vi "DriverStationGetData.vi"   [LabVIEW 2023]
doc: "This VI recieves data from the FRC 4265 Dashboard continuously, in all robot modes. These may include safety overrides, calibration commands, and configuration parameters. However this VI should never include standard driver or manipulator commands."
uses:
  f2972b46-d919-4210-bfdf-d3cf9c7f3ddc.vi
  GlobalDriverStationData.vi
  <vilib>/Rock Robotics/Network Tables/NT Read Number.vi
  <vilib>/Rock Robotics/Network Tables/NT Read Boolean.vi
  GlobalDrivebase.vi
  GlobalPoseAndTargeting.vi
  GlobalShooter.vi
  GlobalElevator.vi
  GlobalDriverStationCommands.vi
  GRNF_Joystick.vi
  <vilib>/Rock Robotics/Network Tables/NT Read Numeric Array.vi
  <vilib>/Rock Robotics/Network Tables/NT Read String.vi
  <vilib>/Utility/xml.llb/Write to XML File(string).vi
types:
  T1 = enum16{"Center", "North", "NorthWest", "West", "SouthWest", "South", "SouthEast", "East", "NorthEast"}
  T2 = typedef "WPI_JoystickDevRef.ctl" = cluster{"Device":T3}
  T3 = typedef "WPI_JoystickDeviceEnum.ctl" = enum16{"USB 0", "USB 1", "USB 2", "USB 3", "USB 4", "USB 5"}
  T4 = typedef "WPI_DriverStationAllianceInfo.ctl" = enum16{"Red", "Blue", "Invalid"}
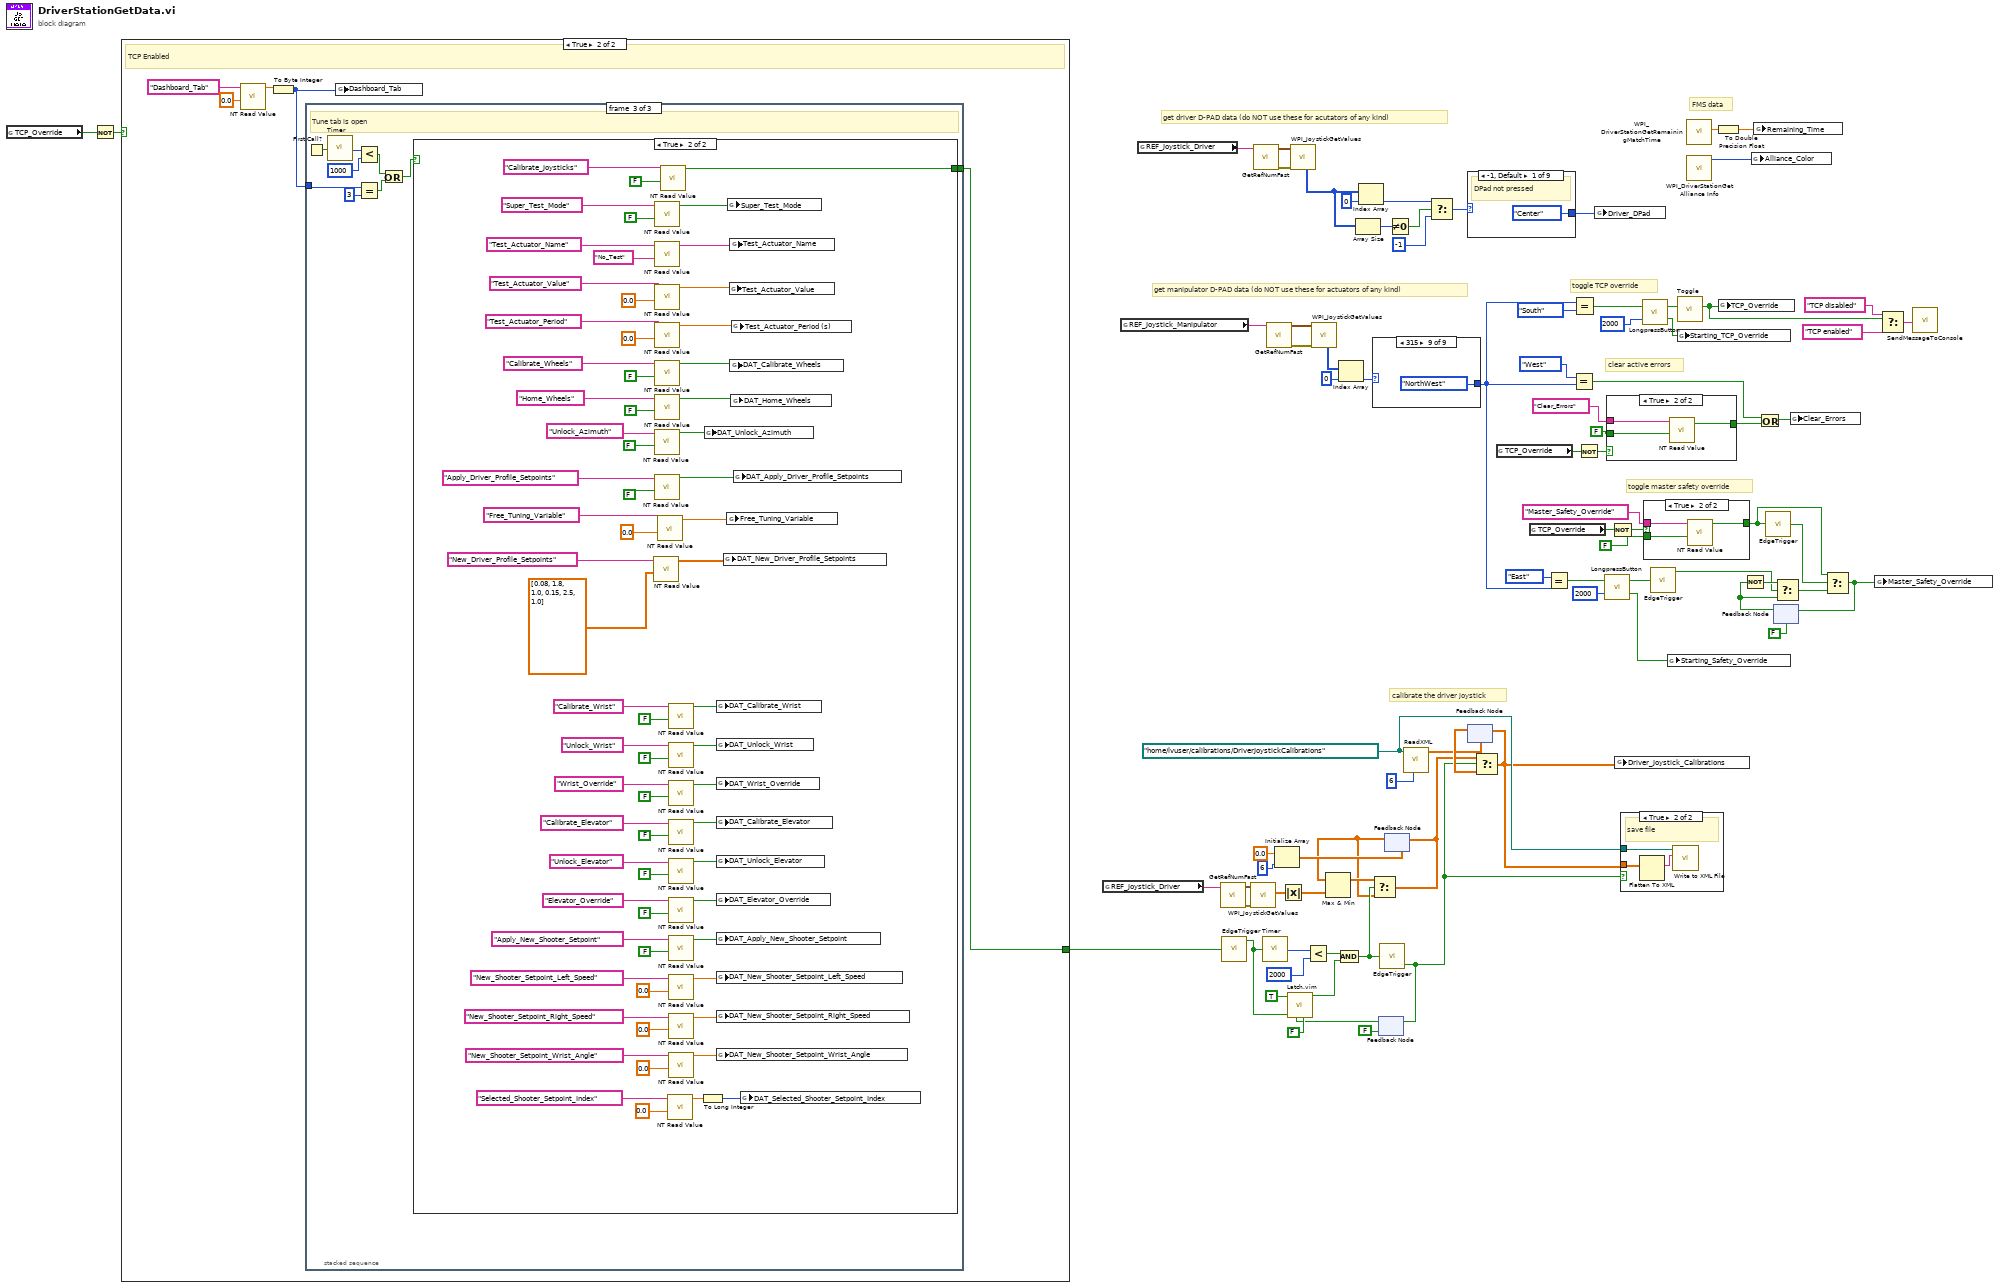
[diagram p0: block diagram]
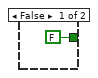
[diagram p2: hidden frame]
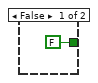
[diagram p3: hidden frame]
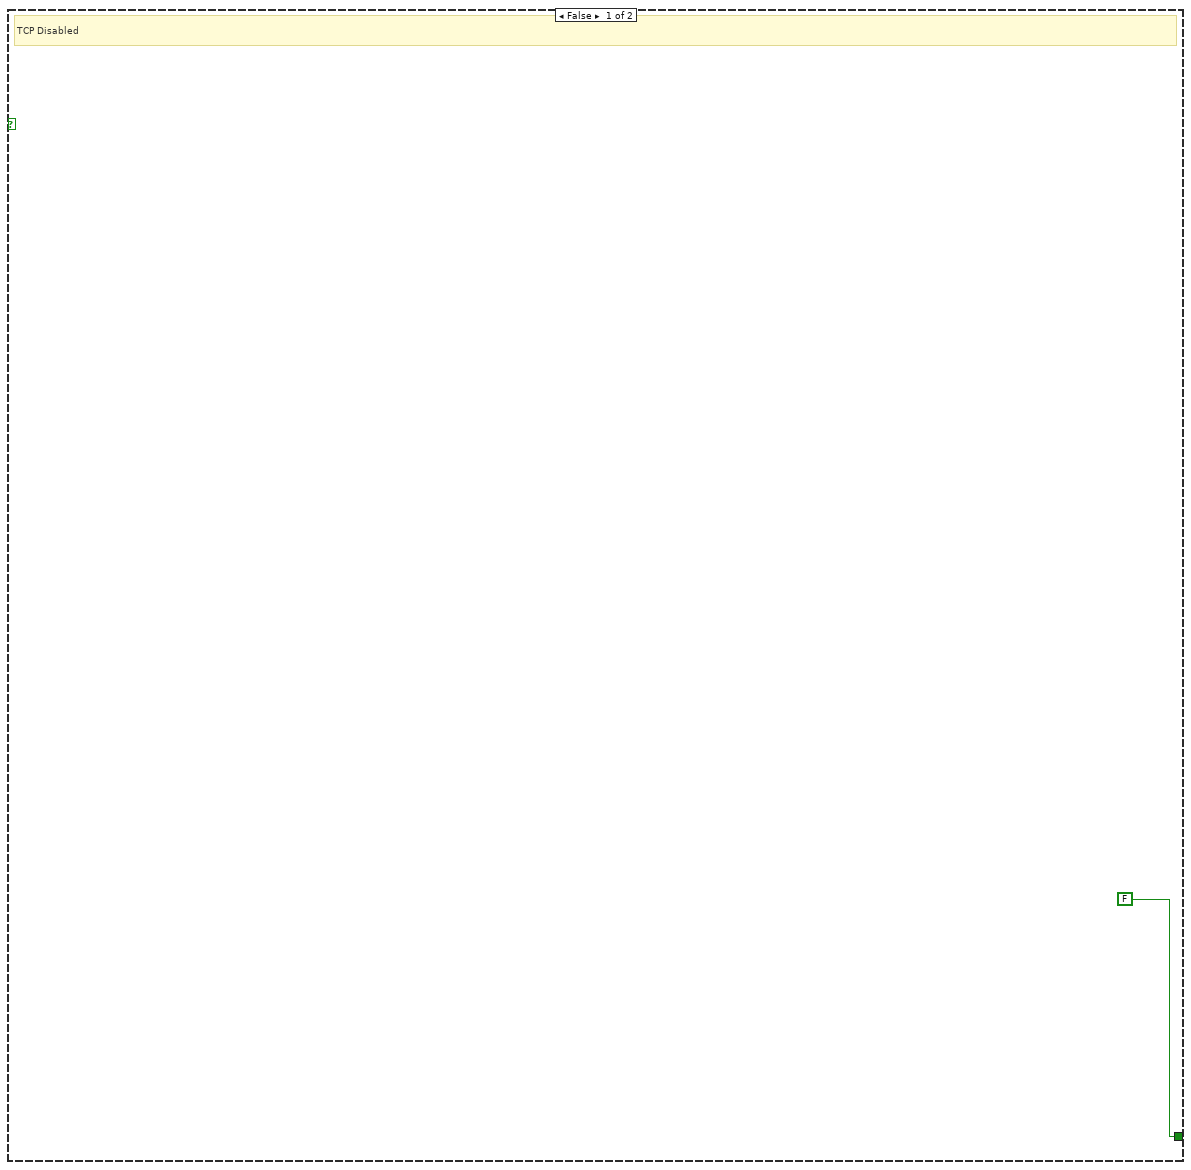
[diagram p4: hidden frame]
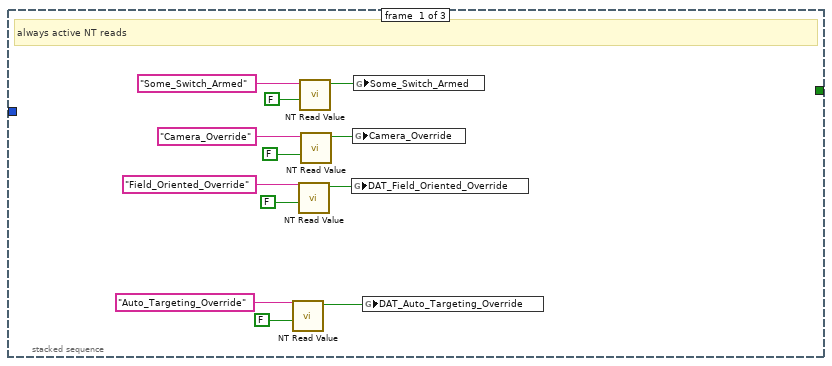
[diagram p5: hidden frame]
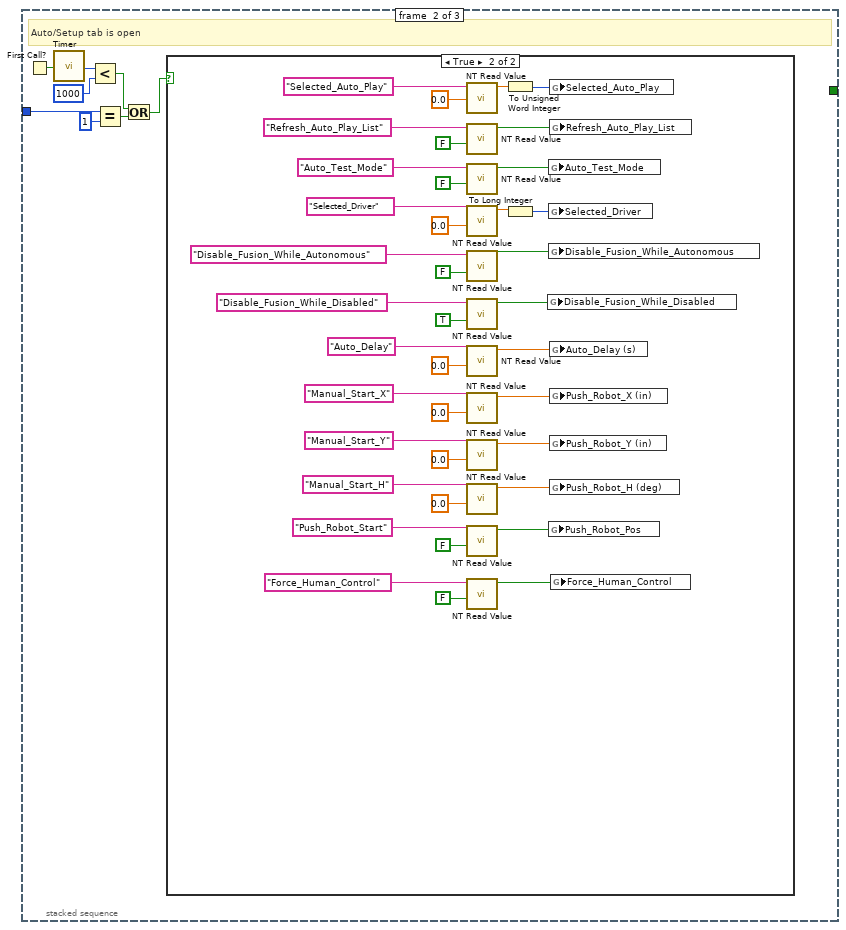
[diagram p6: hidden frame]
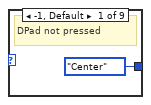
[diagram p9: hidden frame]
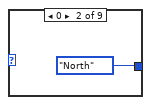
[diagram p10: hidden frame]
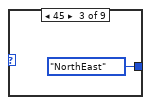
[diagram p11: hidden frame]
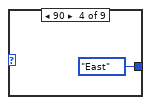
[diagram p12: hidden frame]
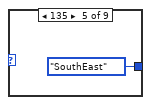
[diagram p13: hidden frame]
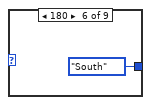
[diagram p14: hidden frame]
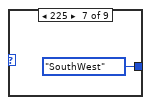
[diagram p15: hidden frame]
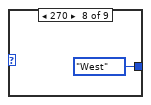
[diagram p16: hidden frame]
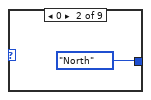
[diagram p17: hidden frame]
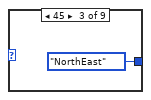
[diagram p18: hidden frame]
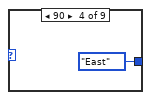
[diagram p19: hidden frame]
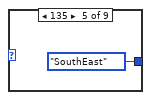
[diagram p20: hidden frame]
diagram:
  w82 = path "/home/lvuser/calibrations/DriverJoystickCalibrations" ("path")
  # "toggle master safety override"
  # "clear active errors"
  # "toggle TCP override"
  # "FMS data"
  # "get manipulator D-PAD data (do NOT use these for actuators of any kind)"
  # "get driver D-PAD data (do NOT use these for acutators of any kind)"
  # "calibrate the driver joystick"
  n1 = global read "GlobalDriverStationData.vi" "TCP_Override"() -> (w15:bool)
  n2 = Not(x=w15) -> (.not. x?=w14:bool)
  n3 = case shown="True" w14 {
    tunnel: [FALSE ("Boolean") w87] -> w26
    frame False {
      # "TCP Disabled"
    }
    frame True {
      # "TCP Enabled"
      n4 = call-poly <vilib>:"NT Read Value.vi"("default value"=0.0 ("Default Value"), "name"="Dashboard_Tab" ("refnum name")) -> ("value"=w89:dbl)  [unwired: 7 in, 2 out]
      n5 = To Byte Integer(number=w89) -> (8bit integer=w88:i8)
      n6 = stacked-sequence {
        tunnel: w88 -> [_ w111 w156]
        tunnel: [_ _ w154] -> w87
        frame #0 {
          # "always active NT reads"
          n7 = call-poly <vilib>:"NT Read Value.vi"("default value"=FALSE ("Default Value"), "name"="Auto_Targeting_Override" ("refnum name")) -> ("value"=w92:bool)  [unwired: 7 in, 2 out]
          n8 = call-poly <vilib>:"NT Read Value.vi"("default value"=FALSE ("Default Value"), "name"="Field_Oriented_Override" ("refnum name")) -> ("value"=w95:bool)  [unwired: 7 in, 2 out]
          n9 = call-poly <vilib>:"NT Read Value.vi"("default value"=FALSE ("Default Value"), "name"="Some_Switch_Armed" ("refnum name")) -> ("value"=w103:bool)  [unwired: 7 in, 2 out]
          n10 = call-poly <vilib>:"NT Read Value.vi"("default value"=FALSE ("Default Value"), "name"="Camera_Override" ("refnum name")) -> ("value"=w100:bool)  [unwired: 7 in, 2 out]
          n11 = global write "GlobalDrivebase.vi" "DAT_Field_Oriented_Override"(w95) -> ()
          n12 = global write "GlobalDriverStationData.vi" "Camera_Override"(w100) -> ()
          n13 = global write "GlobalDriverStationData.vi" "Some_Switch_Armed"(w103) -> ()
          n14 = global write "GlobalDrivebase.vi" "DAT_Auto_Targeting_Override"(w92) -> ()
        }
        frame #1 {
          # "Auto/Setup tab is open"
          n15 = First Call?() -> (First Call?: T/F=w109:bool)
          n16 = call "Timer.vi"("Reset Timer"=w109) -> ("Time (ms)"=w108:u32)
          n17 = Less?(x=w108, y=u32 1000 ("Time threshold (ms)")) -> (x < y?=w106:bool)
          n18 = Equal?(x=w111, y=i8 1) -> (x = y?=w107:bool)
          n19 = Or(x=w106, y=w107) -> (x .or. y?=w105:bool)
          n20 = case shown="True" w105 {
            frame False {
            }
            frame True {
              n21 = call-poly <vilib>:"NT Read Value.vi"("default value"=0.0 ("Default Value"), "name"="Selected_Auto_Play" ("refnum name")) -> ("value"=w138:dbl)  [unwired: 7 in, 2 out]
              n22 = call-poly <vilib>:"NT Read Value.vi"("default value"=FALSE ("Default Value"), "name"="Refresh_Auto_Play_List" ("refnum name")) -> ("value"=w137:bool)  [unwired: 7 in, 2 out]
              n23 = call-poly <vilib>:"NT Read Value.vi"("default value"=FALSE ("Default Value"), "name"="Auto_Test_Mode" ("refnum name")) -> ("value"=w149:bool)  [unwired: 7 in, 2 out]
              n24 = call-poly <vilib>:"NT Read Value.vi"("default value"=0.0 ("Default Value"), "name"="Selected_Driver" ("refnum name")) -> ("value"=w140:dbl)  [unwired: 7 in, 2 out]
              n25 = call-poly <vilib>:"NT Read Value.vi"("default value"=FALSE ("Default Value"), "name"="Disable_Fusion_While_Autonomous" ("refnum name")) -> ("value"=w143:bool)  [unwired: 7 in, 2 out]
              n26 = call-poly <vilib>:"NT Read Value.vi"("default value"=TRUE ("Default Value"), "name"="Disable_Fusion_While_Disabled" ("refnum name")) -> ("value"=w144:bool)  [unwired: 7 in, 2 out]
              n27 = call-poly <vilib>:"NT Read Value.vi"("default value"=0.0 ("Default Value"), "name"="Auto_Delay" ("refnum name")) -> ("value"=w142:dbl)  [unwired: 7 in, 2 out]
              n28 = call-poly <vilib>:"NT Read Value.vi"("default value"=0.0 ("Default Value"), "name"="Manual_Start_X" ("refnum name")) -> ("value"=w145:dbl)  [unwired: 7 in, 2 out]
              n29 = call-poly <vilib>:"NT Read Value.vi"("default value"=0.0 ("Default Value"), "name"="Manual_Start_Y" ("refnum name")) -> ("value"=w146:dbl)  [unwired: 7 in, 2 out]
              n30 = call-poly <vilib>:"NT Read Value.vi"("default value"=0.0 ("Default Value"), "name"="Manual_Start_H" ("refnum name")) -> ("value"=w147:dbl)  [unwired: 7 in, 2 out]
              n31 = call-poly <vilib>:"NT Read Value.vi"("default value"=FALSE ("Default Value"), "name"="Push_Robot_Start" ("refnum name")) -> ("value"=w148:bool)  [unwired: 7 in, 2 out]
              n32 = call-poly <vilib>:"NT Read Value.vi"("default value"=FALSE ("Default Value"), "name"="Force_Human_Control" ("refnum name")) -> ("value"=w114:bool)  [unwired: 7 in, 2 out]
              n33 = To Unsigned Word Integer(number=w138) -> (unsigned 16bit integer=w139:u16)
              n34 = To Long Integer(number=w140) -> (32bit integer=w141:i32)
              n35 = global write "GlobalDriverStationData.vi" "Disable_Fusion_While_Disabled"(w144) -> ()
              n36 = global write "GlobalDriverStationData.vi" "Auto_Test_Mode"(w149) -> ()
              n37 = global write "GlobalDriverStationData.vi" "Selected_Driver"(w141) -> ()
              n38 = global write "GlobalDriverStationData.vi" "Disable_Fusion_While_Autonomous"(w143) -> ()
              n39 = global write "GlobalPoseAndTargeting.vi" "Push_Robot_Pos"(w148) -> ()
              n40 = global write "GlobalDriverStationData.vi" "Selected_Auto_Play"(w139) -> ()
              n41 = global write "GlobalDriverStationData.vi" "Refresh_Auto_Play_List"(w137) -> ()
              n42 = global write "GlobalDriverStationData.vi" "Auto_Delay (s)"(w142) -> ()
              n43 = global write "GlobalPoseAndTargeting.vi" "Push_Robot_X (in)"(w145) -> ()
              n44 = global write "GlobalPoseAndTargeting.vi" "Push_Robot_Y (in)"(w146) -> ()
              n45 = global write "GlobalPoseAndTargeting.vi" "Push_Robot_H (deg)"(w147) -> ()
              n46 = global write "GlobalDriverStationData.vi" "Force_Human_Control"(w114) -> ()
            }
          }
        }
        frame #2 {
          # "Tune tab is open"
          n47 = First Call?() -> (First Call?: T/F=w153:bool)
          n48 = call "Timer.vi"("Reset Timer"=w153) -> ("Time (ms)"=w152:u32)
          n49 = Less?(x=w152, y=u32 1000 ("Time threshold (ms)")) -> (x < y?=w150:bool)
          n50 = Equal?(x=w156, y=i8 3) -> (x = y?=w158:bool)
          n51 = Or(x=w150, y=w158) -> (x .or. y?=w155:bool)
          n52 = case shown="True" w155 {
            tunnel: [_ w200] -> w154
            frame False {
            }
            frame True {
              n53 = call-poly <vilib>:"NT Read Value.vi"("default value"=dbl[] [0.08, 1.8, 1.0, 0.15, 2.5, 1.0] ("Default Value"), "name"="New_Driver_Profile_Setpoints" ("Name")) -> ("value"=w196:dbl[])  [unwired: 7 in, 2 out]
              n54 = call-poly <vilib>:"NT Read Value.vi"("default value"=FALSE ("Default Value"), "name"="Unlock_Azimuth" ("refnum name")) -> ("value"=w193:bool)  [unwired: 7 in, 2 out]
              n55 = call-poly <vilib>:"NT Read Value.vi"("default value"=FALSE ("Default Value"), "name"="Apply_Driver_Profile_Setpoints" ("Name")) -> ("value"=w197:bool)  [unwired: 7 in, 2 out]
              n56 = call-poly <vilib>:"NT Read Value.vi"("default value"=FALSE ("Default Value"), "name"="Super_Test_Mode" ("refnum name")) -> ("value"=w225:bool)  [unwired: 7 in, 2 out]
              n57 = call-poly <vilib>:"NT Read Value.vi"("default value"="No_Test" ("Default Value"), "name"="Test_Actuator_Name" ("refnum name")) -> ("value"=w220:string)  [unwired: 7 in, 2 out]
              n58 = call-poly <vilib>:"NT Read Value.vi"("default value"=0.0 ("Default Value"), "name"="Test_Actuator_Value" ("refnum name")) -> ("value"=w221:dbl)  [unwired: 7 in, 2 out]
              n59 = call-poly <vilib>:"NT Read Value.vi"("default value"=0.0 ("Default Value"), "name"="Test_Actuator_Period" ("refnum name")) -> ("value"=w222:dbl)  [unwired: 7 in, 2 out]
              n60 = call-poly <vilib>:"NT Read Value.vi"("default value"=FALSE ("Default Value"), "name"="Calibrate_Wheels" ("refnum name")) -> ("value"=w199:bool)  [unwired: 7 in, 2 out]
              n61 = call-poly <vilib>:"NT Read Value.vi"("default value"=FALSE ("Default Value"), "name"="Home_Wheels" ("refnum name")) -> ("value"=w198:bool)  [unwired: 7 in, 2 out]
              n62 = call-poly <vilib>:"NT Read Value.vi"("default value"=0.0 ("Default Value"), "name"="Free_Tuning_Variable" ("refnum name")) -> ("value"=w206:dbl)  [unwired: 7 in, 2 out]
              n63 = call-poly <vilib>:"NT Read Value.vi"("default value"=FALSE ("Default Value"), "name"="Calibrate_Joysticks" ("refnum name")) -> ("value"=w200:bool)  [unwired: 7 in, 2 out]
              n64 = call-poly <vilib>:"NT Read Value.vi"("default value"=0.0, "name"="Selected_Shooter_Setpoint_Index" ("refnum name")) -> ("value"=w160:dbl)  [unwired: 7 in, 2 out]
              n65 = call-poly <vilib>:"NT Read Value.vi"("default value"=FALSE ("Default Value"), "name"="Calibrate_Wrist" ("refnum name")) -> ("value"=w190:bool)  [unwired: 7 in, 2 out]
              n66 = call-poly <vilib>:"NT Read Value.vi"("default value"=FALSE ("Default Value"), "name"="Unlock_Wrist" ("refnum name")) -> ("value"=w180:bool)  [unwired: 7 in, 2 out]
              n67 = call-poly <vilib>:"NT Read Value.vi"("default value"=FALSE ("Default Value"), "name"="Wrist_Override" ("refnum name")) -> ("value"=w175:bool)  [unwired: 7 in, 2 out]
              n68 = call-poly <vilib>:"NT Read Value.vi"("default value"=FALSE ("Default Value"), "name"="Calibrate_Elevator" ("refnum name")) -> ("value"=w187:bool)  [unwired: 7 in, 2 out]
              n69 = call-poly <vilib>:"NT Read Value.vi"("default value"=FALSE ("Default Value"), "name"="Unlock_Elevator" ("refnum name")) -> ("value"=w186:bool)  [unwired: 7 in, 2 out]
              n70 = call-poly <vilib>:"NT Read Value.vi"("default value"=FALSE ("Default Value"), "name"="Elevator_Override" ("refnum name")) -> ("value"=w181:bool)  [unwired: 7 in, 2 out]
              n71 = call-poly <vilib>:"NT Read Value.vi"("default value"=FALSE ("Default Value"), "name"="Apply_New_Shooter_Setpoint" ("refnum name")) -> ("value"=w172:bool)  [unwired: 7 in, 2 out]
              n72 = call-poly <vilib>:"NT Read Value.vi"("default value"=0.0, "name"="New_Shooter_Setpoint_Left_Speed" ("refnum name")) -> ("value"=w171:dbl)  [unwired: 7 in, 2 out]
              n73 = call-poly <vilib>:"NT Read Value.vi"("default value"=0.0, "name"="New_Shooter_Setpoint_Right_Speed" ("refnum name")) -> ("value"=w168:dbl)  [unwired: 7 in, 2 out]
              n74 = call-poly <vilib>:"NT Read Value.vi"("default value"=0.0, "name"="New_Shooter_Setpoint_Wrist_Angle" ("refnum name")) -> ("value"=w167:dbl)  [unwired: 7 in, 2 out]
              n75 = To Long Integer(number=w160) -> (32bit integer=w159:i32)
              n76 = global write "GlobalDrivebase.vi" "DAT_Unlock_Azimuth"(w193) -> ()
              n77 = global write "GlobalShooter.vi" "DAT_Calibrate_Wrist"(w190) -> ()
              n78 = global write "GlobalShooter.vi" "DAT_Unlock_Wrist"(w180) -> ()
              n79 = global write "GlobalShooter.vi" "DAT_Wrist_Override"(w175) -> ()
              n80 = global write "GlobalElevator.vi" "DAT_Calibrate_Elevator"(w187) -> ()
              n81 = global write "GlobalElevator.vi" "DAT_Unlock_Elevator"(w186) -> ()
              n82 = global write "GlobalElevator.vi" "DAT_Elevator_Override"(w181) -> ()
              n83 = global write "GlobalShooter.vi" "DAT_Apply_New_Shooter_Setpoint"(w172) -> ()
              n84 = global write "GlobalShooter.vi" "DAT_New_Shooter_Setpoint_Left_Speed"(w171) -> ()
              n85 = global write "GlobalShooter.vi" "DAT_New_Shooter_Setpoint_Right_Speed"(w168) -> ()
              n86 = global write "GlobalShooter.vi" "DAT_New_Shooter_Setpoint_Wrist_Angle"(w167) -> ()
              n87 = global write "GlobalDrivebase.vi" "DAT_New_Driver_Profile_Setpoints"(w196) -> ()
              n88 = global write "GlobalDriverStationData.vi" "Free_Tuning_Variable"(w206) -> ()
              n89 = global write "GlobalDriverStationData.vi" "Super_Test_Mode"(w225) -> ()
              n90 = global write "GlobalDriverStationData.vi" "Test_Actuator_Value"(w221) -> ()
              n91 = global write "GlobalDriverStationData.vi" "Test_Actuator_Name"(w220) -> ()
              n92 = global write "GlobalDrivebase.vi" "DAT_Calibrate_Wheels"(w199) -> ()
              n93 = global write "GlobalDrivebase.vi" "DAT_Home_Wheels"(w198) -> ()
              n94 = global write "GlobalDriverStationData.vi" "Test_Actuator_Period (s)"(w222) -> ()
              n95 = global write "GlobalDrivebase.vi" "DAT_Apply_Driver_Profile_Setpoints"(w197) -> ()
              n96 = global write "GlobalShooter.vi" "DAT_Selected_Shooter_Setpoint_Index"(w159) -> ()
            }
          }
        }
      }
      n97 = global write "GlobalDriverStationData.vi" "Dashboard_Tab"(w88) -> ()
    }
  }
  n98 = global read "GlobalDriverStationCommands.vi" "REF_Joystick_Driver"() -> (w7:string)
  n99 = global read "GlobalDriverStationCommands.vi" "REF_Joystick_Manipulator"() -> (w8:string)
  n100 = global read "GlobalDriverStationCommands.vi" "REF_Joystick_Driver"() -> (w9:string)
  n101 = call-poly "GetRefNumFast.vi"("RefNum Name"=w7) -> ("Error"=w77:errorcluster, "Device Reference"=w78:T2)  [unwired: 5 in]
  n102 = call "EdgeTrigger.vi"("Input Signal"=w26) -> ("Rising Edge Trigger"=w76:bool)  [unwired: 2 out]
  n103 = call <vilib>:"WPI_JoystickGetValues.vi"("error in (no error)"=w77, "JoystickDevRef"=w78) -> ("Axes"=w66:dbl[])  [unwired: 5 in, 4 out]
  n104 = call-poly "GetRefNumFast.vi"("RefNum Name"=w9) -> ("Error"=w56:errorcluster, "Device Reference"=w57:T2)  [unwired: 5 in]
  n105 = call "Timer.vi"("Reset Timer"=w76) -> ("Time (ms)"=w80:u32)
  n106 = call-poly "GetRefNumFast.vi"("RefNum Name"=w8) -> ("Error"=w84:errorcluster, "Device Reference"=w85:T2)  [unwired: 5 in]
  n107 = Initialize Array(0.0 ("element"), 6 ("dimension size")) -> (w59:dbl[])
  n108 = Absolute Value(x=w66) -> (abs(x)=w63:dbl[])
  n109 = call <vilib>:"WPI_JoystickGetValues.vi"("error in (no error)"=w56, "JoystickDevRef"=w57) -> ("POVs"=w6:i16[])  [unwired: 5 in, 4 out]
  n110 = Less?(x=w80, y=u32 2000) -> (x < y?=w73:bool)
  n111 = call <vilib>:"WPI_JoystickGetValues.vi"("error in (no error)"=w84, "JoystickDevRef"=w85) -> ("POVs"=w51:i16[])  [unwired: 5 in, 4 out]
  n112 = Index Array(array=w51, index=0) -> (element=w52:i16)
  n113 = Array Size(array=w6) -> (size(s)=w5:i32)
  n114 = Index Array(array=w6, index=0) -> (element=w4:i16)
  n115 = case shown="315" w52 {
    tunnel: [T1."Center" T1."North" T1."NorthEast" T1."East" T1."SouthEast" T1."South" T1."SouthWest" T1."West" T1."NorthWest"] -> w24
    frame -1, Default {
      # "DPad not pressed"
    }
    frame 0 {
    }
    frame 45 {
    }
    frame 90 {
    }
    frame 135 {
    }
    frame 180 {
    }
    frame 225 {
    }
    frame 270 {
    }
    frame 315 {
    }
  }
  n116 = feedback #1(FALSE ("Falling Edge Trigger")) -> (w70:bool)
  n117 = call "Latch.vim"("Default Value"=FALSE, "Reset"=w70, "Latch Signal"=w76, "Latch Value"=TRUE) -> ("Latched"=w72:bool)  [unwired: 7 in]
  n118 = And(x=w73, y=w72) -> (x .and. y?=w71:bool)
  n119 = call "EdgeTrigger.vi"("Input Signal"=w71) -> ("Falling Edge Trigger"=w68:bool)  [unwired: 2 out]
  n120 = feedback-in #1(w68) -> ()
  n121 = feedback #2(w59) -> (w58:dbl[])
  n122 = Max & Min(x=w58, y=w63) -> (max(x,y)=w65:dbl[])  [unwired: 1 out]
  n123 = Select(t=w65, s=w71, f=w58) -> (s? t:f=w64:dbl[])
  n124 = feedback-in #2(w64) -> ()
  n125 = Not Equal To 0?(x=w5) -> (x != 0?=w3:bool)
  n126 = call "ReadXML.vi"("Default Number of Elements"=6, "File Path (.xml)"=w82) -> ("Data"=w81:dbl[])  [unwired: 8 in, 1 out]
  n127 = Select(t=w4, s=w3, f=i16 -1) -> (s? t:f=w2:i16)
  n128 = case shown="-1, Default" w2 {
    tunnel: [T1."Center" T1."North" T1."NorthEast" T1."East" T1."SouthEast" T1."South" T1."SouthWest" T1."West" T1."NorthWest"] -> w54
    frame -1, Default {
      # "DPad not pressed"
    }
    frame 0 {
    }
    frame 45 {
    }
    frame 90 {
    }
    frame 135 {
    }
    frame 180 {
    }
    frame 225 {
    }
    frame 270 {
    }
    frame 315 {
    }
  }
  n129 = feedback #3(w81) -> (w83:dbl[])
  n130 = Select(t=w64, s=w68, f=w83) -> (s? t:f=w67:dbl[])
  n131 = feedback-in #3(w67) -> ()
  n132 = global read "GlobalDriverStationData.vi" "TCP_Override"() -> (w11:bool)
  n133 = global read "GlobalDriverStationData.vi" "TCP_Override"() -> (w13:bool)
  n134 = Equal?(x=T1."East", y=w24) -> (x = y?=w40:bool)
  n135 = Equal?(x=T1."West", y=w24) -> (x = y?=w42:bool)
  n136 = Equal?(x=w24, y=T1."South") -> (x = y?=w22:bool)
  n137 = Not(x=w11) -> (.not. x?=w10:bool)
  n138 = global write "GlobalDriverStationData.vi" "Driver_DPad"(w54) -> ()
  n139 = call "LongpressButton.vi"("Threshold (ms)"=u32 2000, "Button"=w40) -> ("Starting Press"=w39:bool, "Longpress Button"=w33:bool)
  n140 = case shown="True" w10 {
    tunnel: FALSE ("Default Value") -> [_ w247]
    tunnel: "Clear_Errors" ("refnum name") -> [_ w246]
    tunnel: [FALSE ("Boolean") w245] -> w43
    frame False {
    }
    frame True {
      n141 = call-poly <vilib>:"NT Read Value.vi"("default value"=w247, "name"=w246) -> ("value"=w245:bool)  [unwired: 7 in, 2 out]
    }
  }
  n142 = Not(x=w13) -> (.not. x?=w12:bool)
  n143 = global write "GlobalDriverStationData.vi" "Driver_Joystick_Calibrations"(w67) -> ()
  n144 = case shown="True" w68 {
    tunnel: w82 -> [_ w250]
    tunnel: w67 -> [_ w249]
    frame False {
    }
    frame True {
      # "save file"
      n145 = Flatten To XML(6:w249) -> (2:w248:string)
      n146 = call-poly <vilib>:"Write to XML File.vi"("XML Input"=w248, "XML File Path"=w250) -> ()  [unwired: 7 in, 3 out]
    }
  }
  n147 = call "LongpressButton.vi"("Threshold (ms)"=u32 2000, "Button"=w22) -> ("Starting Press"=w21:bool, "Longpress Button"=w20:bool)
  n148 = case shown="True" w12 {
    tunnel: FALSE ("Default Value") -> [_ w254]
    tunnel: "Master_Safety_Override" ("refnum name") -> [_ w253]
    tunnel: [FALSE ("Boolean") w252] -> w30
    frame False {
    }
    frame True {
      n149 = call-poly <vilib>:"NT Read Value.vi"("default value"=w254, "name"=w253) -> ("value"=w252:bool)  [unwired: 7 in, 2 out]
    }
  }
  n150 = call "EdgeTrigger.vi"("Input Signal"=w33) -> ("Rising Edge Trigger"=w32:bool)  [unwired: 2 out]
  n151 = global write "GlobalDriverStationData.vi" "Starting_Safety_Override"(w39) -> ()
  n152 = call "Toggle.vi"("Trigger"=w20) -> ("New State"=w18:bool)  [unwired: 1 in]
  n153 = global write "GlobalDriverStationData.vi" "Starting_TCP_Override"(w21) -> ()
  n154 = call <vilib>:"WPI_DriverStationGetRemainingMatchTime.vi"() -> ("Match Time(s)"=w50:sgl)  [unwired: 10 in, 1 out]
  n155 = call <vilib>:"WPI_DriverStationGet Alliance Info.vi"() -> ("Alliance"=w48:T4)  [unwired: 6 in, 5 out]
  n156 = To Double Precision Float(number=w50) -> (double precision float=w49:dbl)
  n157 = global write "GlobalDriverStationData.vi" "TCP_Override"(w18) -> ()
  n158 = global write "GlobalDriverStationData.vi" "Alliance_Color"(w48) -> ()
  n159 = global write "GlobalDriverStationData.vi" "Remaining_Time"(w49) -> ()
  n160 = Or(x=w42, y=w43) -> (x .or. y?=w46:bool)
  n161 = call "EdgeTrigger.vi"("Input Signal"=w30) -> ("All Edge Trigger"=w29:bool)  [unwired: 2 out]
  n162 = feedback #4(FALSE ("Initial State")) -> (w35:bool)
  n163 = Not(x=w35) -> (.not. x?=w36:bool)
  n164 = Select(t=w36, s=w32, f=w35) -> (s? t:f=w31:bool)
  n165 = global write "GlobalDriverStationData.vi" "Clear_Errors"(w46) -> ()
  n166 = Select(t=w30, s=w29, f=w31) -> (s? t:f=w28:bool)
  n167 = feedback-in #4(w28) -> ()
  n168 = global write "GlobalDriverStationData.vi" "Master_Safety_Override"(w28) -> ()
  n169 = Select(t="TCP disabled" ("Message String"), s=w18, f="TCP enabled" ("Message String")) -> (s? t:f=w19:string)
  n170 = call "SendMessageToConsole.vi"("Message String"=w19) -> ()  [unwired: 1 in]
